vi "ReportHead.vi"(8 "error in (no error)":errorcluster caption="错误输入（无错误）", 10 "工位名称":string, 11 "产品状态":string) -> (0 "error out":errorcluster caption="错误输出", 3 "report out":refnum<class "NI_report.lvclass"> caption="报表输出")   [LabVIEW 2020]
uses:
  <vilib>/Utility/NIReport.llb/NI_report.lvclass
  <vilib>/addons/_office/_exclsub.llb/font.ctl
  Global_Variable/Global.vi
  <vilib>/addons/_office/NI_ReportGenerationToolkit.lvlib
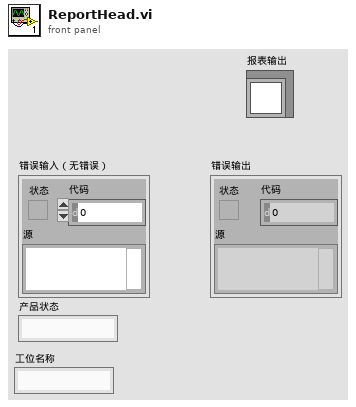
[diagram p1: front panel]
types:
  T1 = cluster{"操作者编号":string, "操作者姓名":string, "操作者权限":string, "联机状态":string, "产品型号":string, "工位名称":string, "产品状态":string}
  T2 = cluster{"top":dbl, "left":dbl, "right":dbl, "bottom":dbl}
  T3 = cluster{"Charset (-1)":i16, "Weight (-1)":i16, "Name":string, "Size":string}
  T4 = cluster{"Italic":enum16{"Italic Unchanged", "Italic On", "Italic Off"}, "Strike Through":enum16{"Strike Through Unchanged", "Strike Through On", "Strike Through Off"}, "Underline":enum16{"Underline Unchanged", "Underline On", "Underline Off"}, "Bold":enum16{"Bold Unchanged", "Bold On", "Bold Off"}}
  T5 = typedef "NI_ReportGenerationToolkit.lvlib/font.ctl" = cluster{"font name":string, "font size":dbl, "bold":u16, "italic":u16, "underline":u16, "strike through":u16, "font color":u32}
  T6 = enum16{"maximized", "minimized", "normal", "no change"}
  T7 = enum16{"Standard Report", "HTML", "Word", "Excel"}
  T8 = cluster{"用户编号":string, "用户名":string, "用户密码(密文)":string, "用户权限":string}
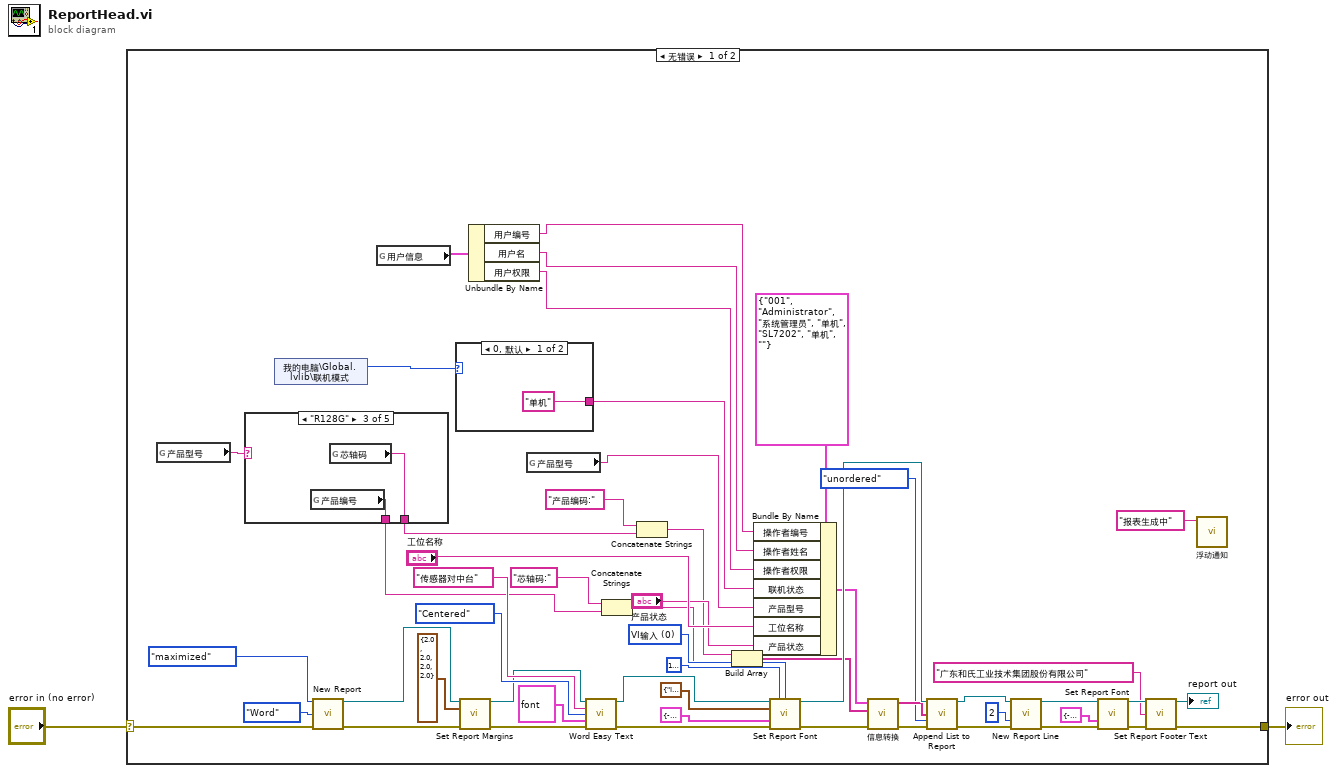
[diagram p0: block diagram]
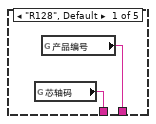
[diagram p2: hidden frame]
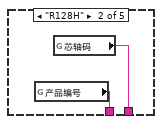
[diagram p3: hidden frame]
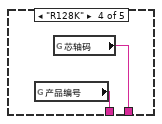
[diagram p4: hidden frame]
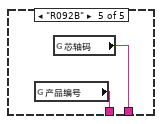
[diagram p5: hidden frame]
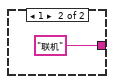
[diagram p6: hidden frame]
diagram:
  n1 = case shown="无错误" "error in (no error)" {
    selector: "error in (no error)" -> [w28 w68]
    tunnel: [w24 w68] -> w1
    frame No Error {
      w48 = u16 0 items=["VI输入", "字体对话框"] ("font settings source")
      n2 = global read "Global.vi" "产品型号"() -> (w6:string)
      n3 = case shown="\"R128G\"" w6 {
        tunnel: [w57 w59 w61 w63 w65] -> w5
        tunnel: [w56 w58 w60 w62 w64] -> w4
        frame "R128", Default {
          n4 = global read "Global.vi" "芯轴码"() -> (w56:string)
          n5 = global read "Global.vi" "产品编号"() -> (w57:string)
        }
        frame "R128H" {
          n6 = global read "Global.vi" "产品编号"() -> (w58:string)
          n7 = global read "Global.vi" "芯轴码"() -> (w59:string)
        }
        frame "R128G" {
          n8 = global read "Global.vi" "产品编号"() -> (w60:string)
          n9 = global read "Global.vi" "芯轴码"() -> (w61:string)
        }
        frame "R128K" {
          n10 = global read "Global.vi" "产品编号"() -> (w62:string)
          n11 = global read "Global.vi" "芯轴码"() -> (w63:string)
        }
        frame "R092B" {
          n12 = global read "Global.vi" "产品编号"() -> (w64:string)
          n13 = global read "Global.vi" "芯轴码"() -> (w65:string)
        }
      }
      n14 = shared-variable "我的电脑\\Global.lvlib\\联机模式"() -> (w22:i16)  [unwired: 1 in, 1 out]
      n15 = call <vilib>:"New Report.vi"("window state (normal)"=T6."maximized", "report type"=T7."Word", "error in (no error)"=w28) -> ("report out"=w41:refnum<class "NI_report.lvclass">, "error out"=w38:errorcluster)  [unwired: 11 in]
      n16 = global read "Global.vi" "用户信息"() -> (w12:T8)
      n17 = case shown="0, 默认" w22 {
        tunnel: ["单机" "联机"] -> w21
        frame 0, Default {
        }
        frame 1 {
        }
      }
      n18 = call-dynamic "Set Report Margins.vi"("report in"=w41, "margins (1.00)"=T2 {"top"=2.0, "left"=2.0, "right"=2.0, "bottom"=2.0}, "error in (no error)"=w38) -> ("report out"=w40:refnum<class "NI_report.lvclass">, "error out"=w39:errorcluster)  [unwired: 10 in, 1 out]
      n19 = Unbundle By Name(w12) -> ("用户编号"=w11:string, "用户名"=w10:string, "用户权限"=w9:string)
      n20 = global read "Global.vi" "产品型号"() -> (w15:string)
      n21 = call <vilib>:"Word Easy Text.vi"("report in"=w40, "text"="传感器对中台", "alignment (left)"=enum16{"Left", "Centered", "Right", "Justify"}."Centered", "font"=T5 {"font name"="楷体", "font size"=26.0, "bold"=1, "italic"=2, "underline"=2, "strike through"=2, "font color"=16777228}, "error in (no error)"=w39) -> ("report out"=w50:refnum<class "NI_report.lvclass">, "error out"=w49:errorcluster)  [unwired: 8 in, 1 out]
      n22 = Concatenate Strings("芯轴码:", w4) -> (w7:string)
      n23 = Concatenate Strings("产品编码:", w5) -> (w3:string)
      n24 = Build Array(w3, w7) -> (w17:string[])
      n25 = Bundle By Name(cluster=T1 {"操作者编号"="001", "操作者姓名"="Administrator", "操作者权限"="系统管理员", "联机状态"="单机", "产品型号"="SL7202", "工位名称"="单机", "产品状态"=""} ("测试信息"), "操作者编号"=w11, "操作者姓名"=w10, "操作者权限"=w9, "联机状态"=w21, "产品型号"=w15, "工位名称"="工位名称", "产品状态"="产品状态") -> (w19:T1)
      n26 = call-dynamic "Set Report Font.vi"("report in"=w50, "text color (unchanged)"=u32 16777224, "font settings source (VI Inputs)"=w48, "text options"=T4 {"Italic"=enum."Italic Off", "Strike Through"=enum."Strike Through Unchanged", "Underline"=enum."Underline Off", "Bold"=enum."Bold Off"}, "font settings"=T3 {"Charset (-1)"=-1, "Weight (-1)"=-1, "Name"="微软雅黑 Light", "Size"="12 "}, "error in (no error)"=w49) -> ("report out"=w36:refnum<class "NI_report.lvclass">, "error out"=w27:errorcluster)  [unwired: 7 in, 1 out]
      n27 = call "信息转换.vi"("错误输入（无错误）"=w27, "追溯码"=w17, "测试信息"=w19) -> ("错误输出"=w26:errorcluster, "信息输出"=w29:string[])  [unwired: 7 in]
      n28 = call-dynamic "Append List to Report.vi"("report in"=w36, "list elements"=w29, "list type (ordered)"=enum16{"unordered", "ordered"}."unordered", "error in (no error)"=w26) -> ("report out"=w31:refnum<class "NI_report.lvclass">, "error out"=w30:errorcluster)  [unwired: 8 in, 2 out]
      n29 = call-dynamic "New Report Line.vi"("report in"=w31, "number of lines (1)"=2, "error in (no error)"=w30) -> ("report out"=w34:refnum<class "NI_report.lvclass">, "error out"=w35:errorcluster)  [unwired: 11 in]
      n30 = call-dynamic "Set Report Font.vi"("report in"=w34, "font settings"=T3 {"Charset (-1)"=-1, "Weight (-1)"=-1, "Name"="楷体", "Size"="9 "}, "error in (no error)"=w35) -> ("report out"=w45:refnum<class "NI_report.lvclass">, "error out"=w44:errorcluster)  [unwired: 10 in, 1 out]
      n31 = call-dynamic "Set Report Footer Text.vi"("report in"=w45, "center footer text"="广东和氏工业技术集团股份有限公司", "error in (no error)"=w44) -> ("report out"=→"report out":refnum<class "NI_report.lvclass">, "error out"=w24:errorcluster)  [unwired: 11 in]
      n32 = call "浮动通知.vi"("通知内容"="报表生成中" ("Status")) -> ()  [unwired: 11 in]
    }
    frame Error {
    }
  }
  "error out" <- w1
